vi "Configure Hardware Finite.vi"(8 "error in (no error)":errorcluster caption="错误输入（无错误）", 11 "Hardware Resources in":T1={"电压读取设置"={"DAQmx Channel"="", "Max Input"=0.0, "Min Input"=0.0, "Sample Rate"=0.0, "Sample Number"=0, "DAQmx Task"="", "device in"=""}, "角度传感器设置"={"counter"="Dev1/ctr0", "units"=10146, "分辨率"=0, "初始角度"=0.0, "DecodingType"=10092, "A相端口"="/Dev1/PFI8", "B相端口"="/Dev1/PFI8", "task in"=""}} caption="硬件资源输入" {"角度传感器设置"."DecodingType" items=["X1"=10090, "X2"=10091, "X4"=10092, "Two Pulse Counting"=10313]; "角度传感器设置"."units" items=["Degrees"=10146, "Radians"=10273, "Ticks"=10304, "From Custom Scale"=10065]}) -> (0 "error out":errorcluster caption="错误输出", 3 "Hardware Resources out":T1={"电压读取设置"={"DAQmx Channel"="", "Max Input"=0.0, "Min Input"=0.0, "Sample Rate"=0.0, "Sample Number"=0, "DAQmx Task"="", "device in"=""}, "角度传感器设置"={"counter"="Dev1/ctr0", "units"=10146, "分辨率"=0, "初始角度"=0.0, "DecodingType"=10092, "A相端口"="/Dev1/PFI8", "B相端口"="/Dev1/PFI8", "task in"=""}} caption="硬件资源输出" {"角度传感器设置"."DecodingType" items=["X1"=10090, "X2"=10091, "X4"=10092, "Two Pulse Counting"=10313]; "角度传感器设置"."units" items=["Degrees"=10146, "Radians"=10273, "Ticks"=10304, "From Custom Scale"=10065]})   [LabVIEW 2015, in "Acquisition.lvlib"]
doc: "配置硬件。"
uses:
  Acquisition.lvlib
  Hardware Configuration.ctl
  <vilib>/DAQmx/create/channels.llb/DAQmx Create Channel (CI-Position-Angular Encoder).vi
  <vilib>/DAQmx/create/channels.llb/DAQmx Create Channel (AI-Voltage-Basic).vi
  <vilib>/DAQmx/configure/timing.llb/DAQmx Timing (Sample Clock).vi
  <resource>/objmgr/daqmx.rc
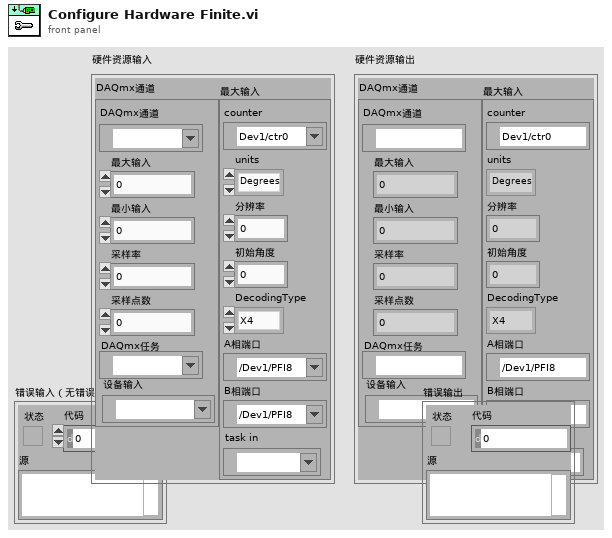
[diagram p1: front panel]
types:
  T1 = typedef "Acquisition.lvlib/Hardware Configuration.ctl" = cluster{"电压读取设置":cluster{"DAQmx Channel":tag, "Max Input":dbl, "Min Input":dbl, "Sample Rate":dbl, "Sample Number":i32, "DAQmx Task":refnum<k21>, "device in":tag}, "角度传感器设置":cluster{"counter":tag, "units":i32, "分辨率":i32, "初始角度":dbl, "DecodingType":i32, "A相端口":tag, "B相端口":tag, "task in":refnum<k21>}}
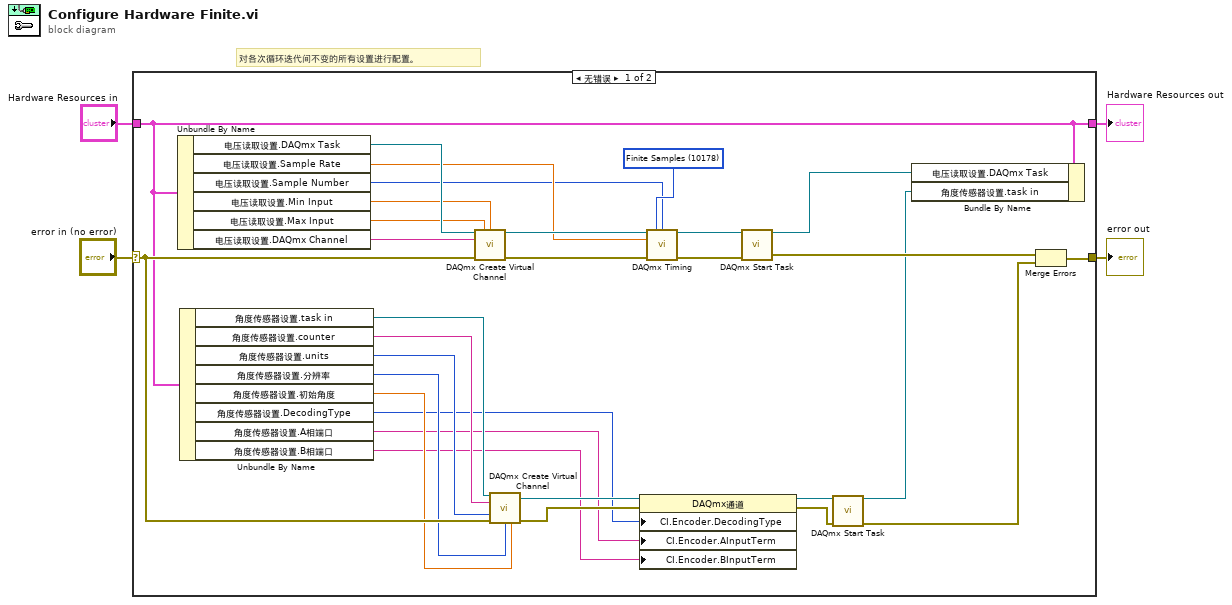
[diagram p0: block diagram]
diagram:
  # "对各次循环迭代间不变的所有设置进行配置。"
  n1 = case shown="无错误" "error in (no error)" {
    selector: "error in (no error)" -> [w20 w35]
    tunnel: [w10 w35] -> w3
    tunnel: "Hardware Resources in" -> [w7 w36]
    tunnel: [w7 w36] -> w1
    frame No Error {
      w28 = 10178 items=["Finite Samples"=10178, "Continuous Samples"=10123, "Hardware Timed Single Point"=12522] ("sample mode")
      n2 = Unbundle By Name(w7) -> ("电压读取设置.DAQmx Task"=w34:refnum<k21>, "电压读取设置.Sample Rate"=w27:dbl, "电压读取设置.Sample Number"=w24:i32, "电压读取设置.Min Input"=w31:dbl, "电压读取设置.Max Input"=w32:dbl, "电压读取设置.DAQmx Channel"=w33:tag)
      n3 = Unbundle By Name(w7) -> ("角度传感器设置.task in"=w23:refnum<k21>, "角度传感器设置.counter"=w22:tag, "角度传感器设置.units"=w21:i32, "角度传感器设置.分辨率"=w19:i32, "角度传感器设置.初始角度"=w18:dbl, "角度传感器设置.DecodingType"=w15:i32, "角度传感器设置.A相端口"=w14:tag, "角度传感器设置.B相端口"=w13:tag)
      n4 = call-poly <vilib>:"DAQmx Create Virtual Channel.vi"("task in"=w34, "maximum value"=w32, "minimum value"=w31, "physical channels"=w33, "error in"=w20) -> ("task out"=w30:refnum<k21>, "error out"=w29:errorcluster)  [unwired: 9 in]
      n5 = call-poly <vilib>:"DAQmx Create Virtual Channel.vi"("task in"=w23, "counter"=w22, "units"=w21, "error in"=w20, "pulses per revolution"=w19, "initial angle"=w18) -> ("task out"=w17:refnum<k21>, "error out"=w16:errorcluster)  [unwired: 8 in]
      n6 = property class="DAQmx通道"(reference=w17, error in=w16, "CI.Encoder.DecodingType"=w15, "CI.Encoder.AInputTerm"=w14, "CI.Encoder.BInputTerm"=w13) -> (reference out=w12:refnum<k21>, error out=w11:errorcluster)
      n7 = call-poly <vilib>:"DAQmx Timing.vi"("task/channels in"=w30, "sample mode"=w28, "samples per channel"=w24, "rate"=w27, "error in"=w29) -> ("task out"=w25:refnum<k21>, "error out"=w26:errorcluster)  [unwired: 9 in]
      n8 = call <vilib>:"DAQmx Start Task.vi"("task/channels in"=w25, "error in"=w26) -> ("task out"=w6:refnum<k21>, "error out"=w9:errorcluster)  [unwired: 12 in]
      n9 = call <vilib>:"DAQmx Start Task.vi"("task/channels in"=w12, "error in"=w11) -> ("task out"=w5:refnum<k21>, "error out"=w8:errorcluster)  [unwired: 12 in]
      n10 = Bundle By Name(cluster=w7, "电压读取设置.DAQmx Task"=w6, "角度传感器设置.task in"=w5) -> ()  [unwired: 1 out]
      n11 = Merge Errors(w9, w8) -> (w10:errorcluster)
    }
    frame Error {
    }
  }
  "Hardware Resources out" <- w1
  "error out" <- w3
